vi "DAQmx Create Channel (AI-Temperature-Built-in Sensor).vi"(0 "task in":refnum<k21>, 5 "physical channels":tag, 7 "name to assign":string, 9 "units":i32(ring)=10143 items=["Deg C"=10143, "Deg F"=10144, "Kelvins"=10325, "Deg R"=10145, "From Custom Scale"=10065], 11 "error in":errorcluster) -> (4 "task out":refnum<k21>, 15 "error out":errorcluster)   [LabVIEW 2011]
doc: "Creates channel(s) that use the built-in sensor of a terminal block or device to measure temperature. On SCXI modules, for example, the built-in sensor could be the CJC sensor."
uses:
  C:/Program Files/National Instruments/LabVIEW 2011/resource/objmgr/daqmx.rc
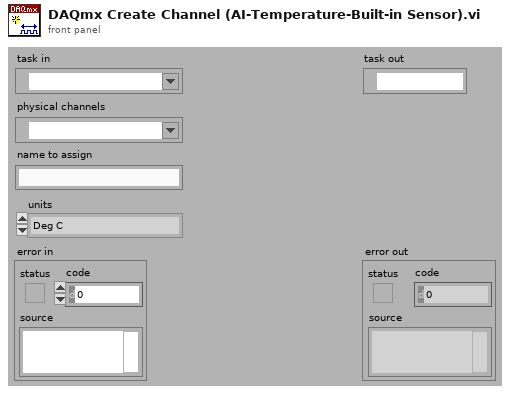
[diagram p1: front panel]
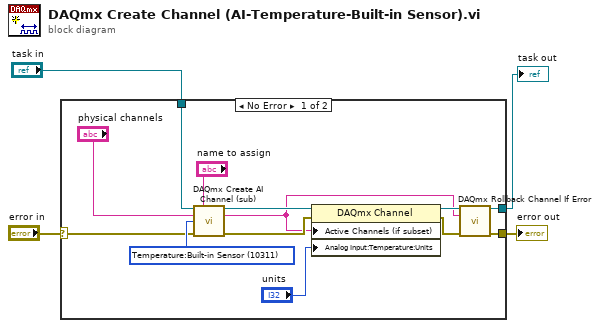
[diagram p0: block diagram]
diagram:
  n1 = case shown="No Error" "error in" {
    selector: "error in" -> [w12 w18]
    tunnel: [w7 w18] -> w4
    tunnel: "task in" -> [w17 w19]
    tunnel: [w9 w19] -> w1
    frame No Error {
      w13 = 10311 items=["Voltage"=10322, "Current"=10134, "More:Voltage:Custom with Excitation"=10323, "More:Current:Custom with Excitation"=10136, "Frequency"=10181, "Period"=10257, "Resistance"=10278, "Temperature:Thermocouple"=10303, "Temperature:Thermistor"=10302, "Temperature:RTD"=10301, "Temperature:Built-in Sensor"=10311, "Strain Gage"=10300] ("measurement type")
      n2 = call "DAQmx Create AI Channel (sub).vi"("task in"=w17, "virtual channel name"="name to assign", "physical channel name"="physical channels", "measurement type"=w13, "error in"=w12) -> ("task out"=w10:refnum<k21>, "channel names"=w5:string, "error out"=w15:errorcluster)  [unwired: 2 in, 6 out]
      n3 = property class="DAQmx Channel"(reference=w10, error in=w15, "Active Channels (if subset)"=w5, "Analog Input:Temperature:Units"="units") -> (reference out=w8:refnum<k21>, error out=w6:errorcluster)
      n4 = call "DAQmx Rollback Channel If Error.vi"("task in"=w8, "channel names"=w5, "error in"=w6) -> ("task out"=w9:refnum<k21>, "error out"=w7:errorcluster)  [unwired: 11 out]
    }
    frame Error {
    }
  }
  "error out" <- w4
  "task out" <- w1
